vi "write.vi"() -> ()   [LabVIEW 2015]
uses:
  <vilib>/Instr/_visa.llb/VISA Configure Serial Port (Instr).vi
panel:
  in  "VISA resource name":refnum<visa-resource-name>
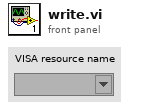
[diagram p1: front panel]
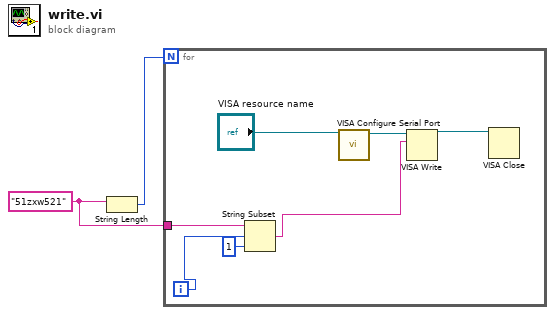
[diagram p0: block diagram]
diagram:
  w1 = "51zxw521" ("write buffer")
  n1 = String Length(string=w1) -> (length=w2:i32)
  n2 = for {
    N: w2 -> [_]
    tunnel: w1 -> [w6]
    i -> [w5]
    n3 = String Subset(string=w6, offset (0)=w5, length (rest)=1 ("length (rest)")) -> (substring=w3:string)
    n4 = call-poly "VISA Configure Serial Port"("VISA resource name"="VISA resource name") -> ("VISA resource name out"=w8:refnum<visa-resource-name>)  [unwired: 13 in, 1 out]
    n5 = VISA Write(VISA resource name=w8, write buffer=w3) -> (VISA resource name out=w7:refnum<visa-resource-name>)  [unwired: 1 in, 2 out]
    n6 = VISA Close(VISA resource name=w7) -> ()  [unwired: 1 in, 1 out]
  }
